vi "current initial.vi"(8 "error in":errorcluster caption="에러 입력", 11 "Current Sourcing":dbl=0.004) -> (0 "error out":errorcluster caption="에러 출력", 1 "Current 배열":dbl[](array[numeric]), 3 "task out":refnum<k21> caption="태스크 출력")   [LabVIEW 2013]
uses:
  <vilib>/DAQmx/create/channels.llb/DAQmx Create Channel (AO-Current-Basic).vi
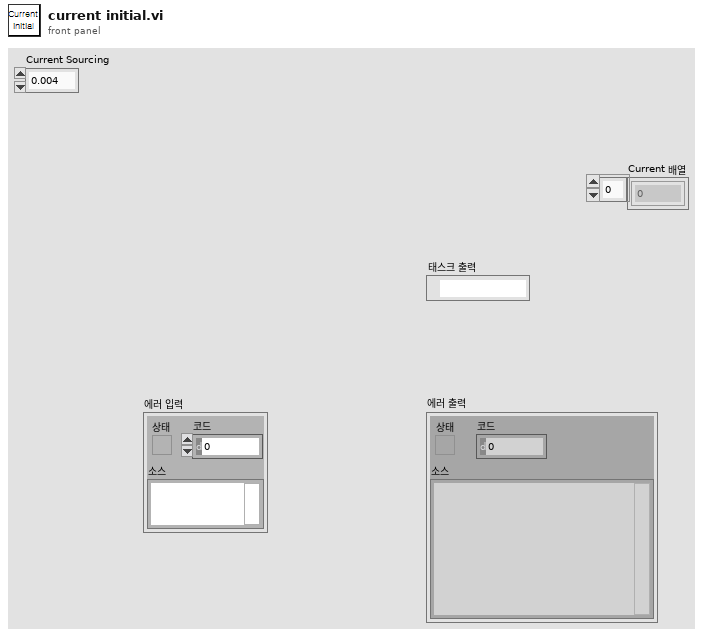
[diagram p1: front panel]
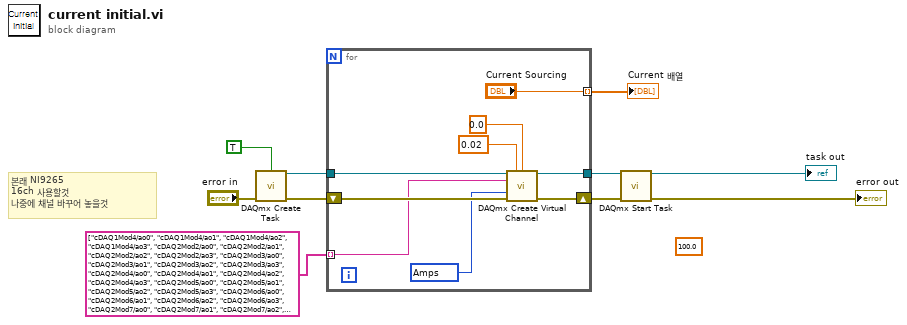
[diagram p0: block diagram]
diagram:
  (unwired) 100.0 ("timeout")
  # "본래 NI9265 \n16ch 사용할것\n나중에 채널 바꾸어 놓을것"
  n1 = call <vilib>:"DAQmx Create Task.vi"("auto cleanup"=TRUE, "error in"="error in") -> ("task out"=w8:refnum<k21>, "error out"=w10:errorcluster)  [unwired: 12 in]
  n2 = for "For 루프" {
    tunnel: w8 -> [w19]
    tunnel: [w17] -> w6
    shift-right: [w16] -> w5
    shift-left: w10 -> [w18]
    tunnel: tag[] ["cDAQ1Mod4/ao0", "cDAQ1Mod4/ao1", "cDAQ1Mod4/ao2", "cDAQ1Mod4/ao3", "cDAQ2Mod2/ao0", "cDAQ2Mod2/ao1", "cDAQ2Mod2/ao2", "cDAQ2Mod2/ao3", "cDAQ2Mod3/ao0", "cDAQ2Mod3/ao1", "cDAQ2Mod3/ao2", "cDAQ2Mod3/ao3", "cDAQ2Mod4/ao0", "cDAQ2Mod4/ao1", "cDAQ2Mod4/ao2", "cDAQ2Mod4/ao3", "cDAQ2Mod5/ao0", "cDAQ2Mod5/ao1", "cDAQ2Mod5/ao2", "cDAQ2Mod5/ao3", "cDAQ2Mod6/ao0", "cDAQ2Mod6/ao1", "cDAQ2Mod6/ao2", "cDAQ2Mod6/ao3", "cDAQ2Mod7/ao0", "cDAQ2Mod7/ao1", "cDAQ2Mod7/ao2", "cDAQ2Mod7/ao3", "cDAQ2Mod8/ao0", "cDAQ2Mod8/ao1", "cDAQ2Mod8/ao2", "cDAQ2Mod8/ao3", "cDAQ3Mod1/ao0", "cDAQ3Mod1/ao1", "cDAQ3Mod1/ao2", "cDAQ3Mod1/ao3", "cDAQ3Mod2/ao0", "cDAQ3Mod2/ao1", "cDAQ3Mod2/ao2", "cDAQ3Mod2/ao3"] -> [w12] mode=indexing
    tunnel: ["Current Sourcing"] -> w2 mode=indexing
    w13 = 10342 items=["Amps"=10342, "사용자 스케일로부터"=10065] ("units")
    n3 = call-poly <vilib>:"DAQmx Create Virtual Channel.vi"("task in"=w19, "maximum value"=0.02, "minimum value"=0.0, "physical channels"=w12, "units"=w13, "error in"=w18) -> ("task out"=w17:refnum<k21>, "error out"=w16:errorcluster)  [unwired: 8 in]
  }
  "Current 배열" <- w2
  n4 = call <vilib>:"DAQmx Start Task.vi"("task/channels in"=w6, "error in"=w5) -> ("task out"=→"task out":refnum<k21>, "error out"=→"error out":errorcluster)  [unwired: 12 in]
